vi "IOOperation.vi"(8 "error in":errorcluster caption="错误输入", 9 "Value":string, 10 "Channel":string, 11 "Com":refnum<visa-resource-name>) -> (0 "error out":errorcluster caption="错误输出", 2 "ComOut":refnum<visa-resource-name>, 3 "DOStatus":bool)   [LabVIEW 2013]
uses:
  GlobValue.vi
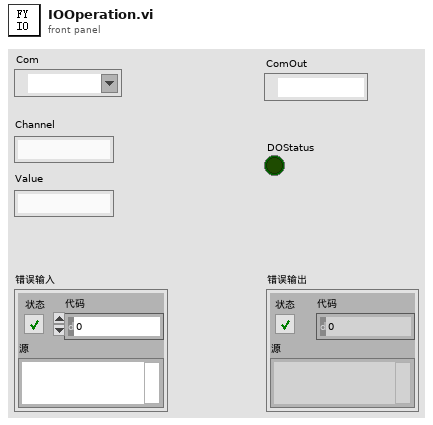
[diagram p1: front panel]
types:
  T1 = typedef "IOConfig.ctl" = cluster{"DO":string[][], "DI":string[][]}
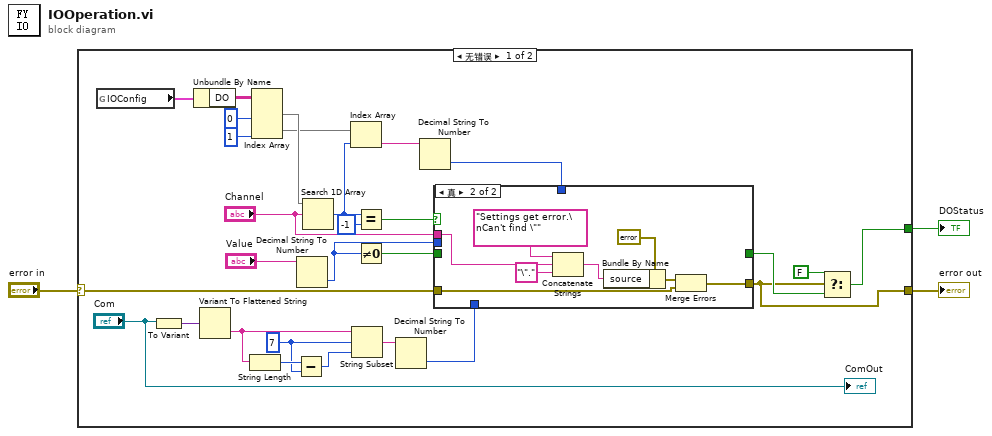
[diagram p0: block diagram]
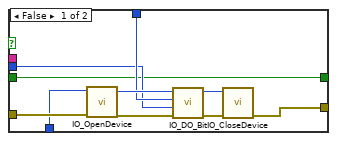
[diagram p2: hidden frame]
diagram:
  n1 = case shown="无错误" "error in" {
    selector: "error in" -> [w21 w50]
    tunnel: [w5 w50] -> w2
    tunnel: [w4 _] -> w1
    frame No Error {
      w15 = 7 ("y")
      n2 = global read "GlobValue.vi" "IOConfig"() -> (w31:T1)
      n3 = To Variant(anything="Com") -> (Variant=w18:variant)
      n4 = Unbundle By Name(w31) -> ("DO"=w30:string[][])
      n5 = Variant To Flattened String(Variant=w18) -> (data string=w14:string)  [unwired: 1 out]
      n6 = String Length(string=w14) -> (length=w17:i32)
      n7 = Index Array(array=w30, index (col) #1=0 ("禁用的索引 (列)"), index (col) #2=1 ("禁用的索引 (列)")) -> (element #1=w28:string[], element #2=w26:string[])  [unwired: 2 in]
      n8 = Subtract(x=w17, y=w15) -> (x-y=w16:i32)
      n9 = Decimal String To Number(string="Value") -> (number=w9:i32)  [unwired: 2 in, 1 out]
      n10 = Search 1D Array(1D array=w28, element="Channel") -> (index of element=w25:i32)  [unwired: 1 in]
      n11 = Index Array(array=w26, index=w25) -> (element=w20:string)
      n12 = String Subset(string=w14, offset (0)=w15, length (rest)=w16) -> (substring=w13:string)
      n13 = Equal?(x=w25, y=-1) -> (x = y?=w23:bool)
      n14 = Not Equal To 0?(x=w9) -> (x != 0?=w8:bool)
      n15 = Decimal String To Number(string=w13) -> (number=w12:i32)  [unwired: 2 in, 1 out]
      n16 = Decimal String To Number(string=w20) -> (number=w11:i32)  [unwired: 2 in, 1 out]
      n17 = case shown="真" w23 {
        tunnel: "Channel" -> [_ w45]
        tunnel: w21 -> [w41 w44]
        tunnel: [w34 w43] -> w5
        tunnel: w12 -> [w40 _]
        tunnel: w11 -> [w37 _]
        tunnel: w9 -> [w36 _]
        tunnel: w8 -> [w32 _]
        tunnel: [w32 _] -> w7
        frame False {
          n18 = call "IO_OpenDevice.vi"("error in"=w41, "ComNum"=w40) -> ("error out"=w39:errorcluster, "hDevice"=w38:u32)  [unwired: 4 in]
          n19 = call "IO_DO_Bit.vi"("error in"=w39, "dodata"=w36, "doch"=w37, "hDevice"=w38) -> ("error out"=w35:errorcluster, "hDeviceOut"=w33:u32)  [unwired: 1 in, 1 out]
          n20 = call "IO_CloseDevice.vi"("error in"=w35, "hDevice"=w33) -> ("error out"=w34:errorcluster)  [unwired: 3 in, 2 out]
        }
        frame True {
          n21 = Concatenate Strings("Settings get error.\nCan't find \"" ("message"), w45, "\"." ("string")) -> (w48:string)
          n22 = Bundle By Name(cluster=errorcluster {"status"=TRUE, "code"=5000, "source"=""} ("error in 1 (no error)"), "source"=w48) -> (w47:errorcluster)
          n23 = Merge Errors(w47, w44) -> (w43:errorcluster)
        }
      }
      n24 = Select(t=FALSE, s=w5, f=w7) -> (s? t:f=w4:bool)
      "ComOut" <- "Com"
    }
    frame Error {
    }
  }
  "error out" <- w2
  "DOStatus" <- w1
